vi "TDK工况电流1.vi"() -> ()   [LabVIEW 2020]
uses:
  <vilib>/Utility/file.llb/Read Delimited Spreadsheet (DBL).vi
  <instrlib>/TDK-Lambda G Series/TDK-Lambda G Series.lvlib
panel:
  in  "循环次数":i32
  out "XY Graph":cluster{"Y":dbl[], "Y":dbl[]}[](graph) caption="XY图"
  in  "VISA resource name":refnum<visa-resource-name>
  in  "file path (dialog if empty)":path caption="文件路径 （空时为对话框）"
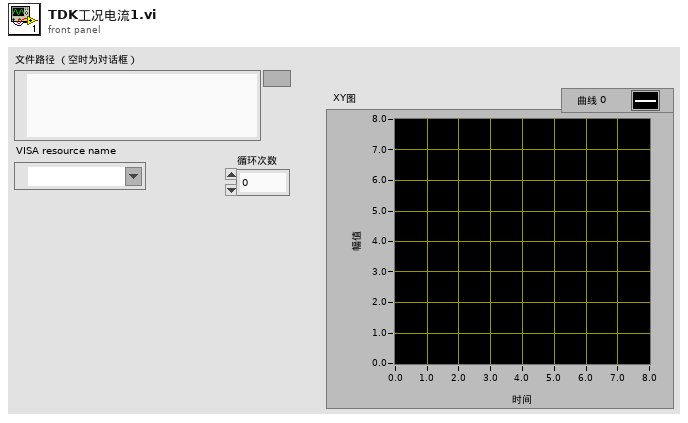
[diagram p1: front panel]
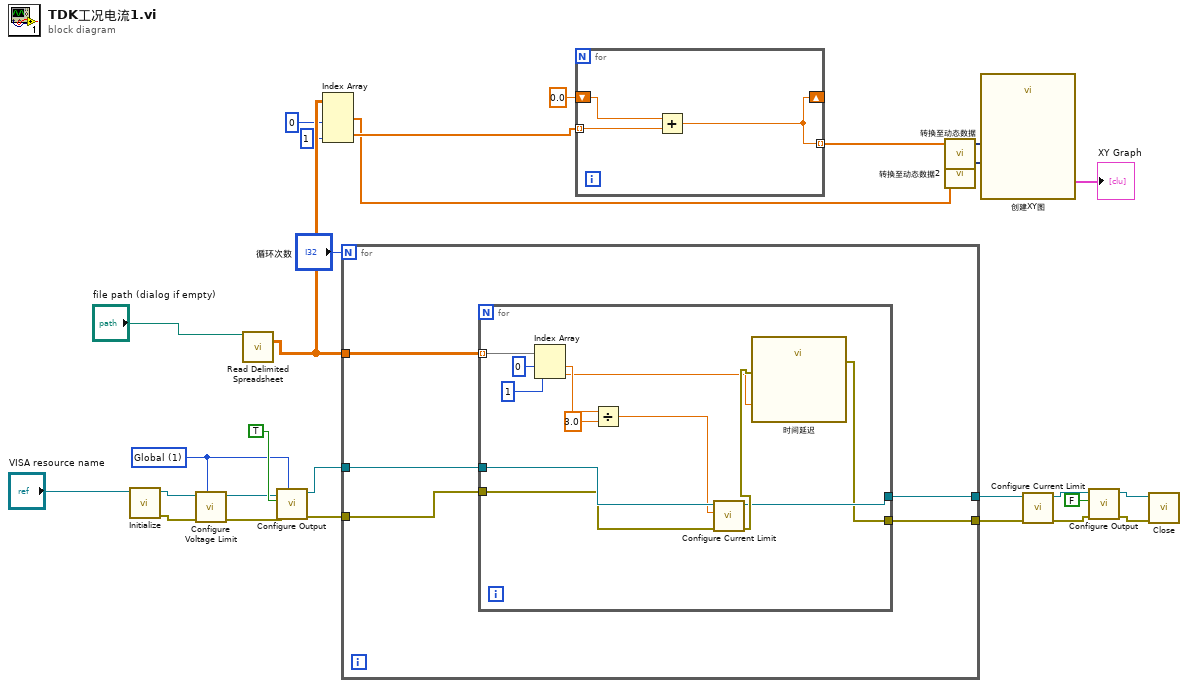
[diagram p0: block diagram]
diagram:
  w23 = u16 1 items=["Single", "Global"] ("Globalize (0: Single)")
  n1 = call <instrlib>:"Initialize.vi"("VISA resource name"="VISA resource name") -> ("error out"=w25:errorcluster, "VISA resource name out"=w22:refnum<visa-resource-name>)  [unwired: 9 in]
  n2 = call <instrlib>:"Configure Voltage Limit.vi"("Globalize (0: Single)"=w23, "error in (no error)"=w25, "VISA resource name"=w22) -> ("error out"=w24:errorcluster, "VISA resource name out"=w21:refnum<visa-resource-name>)  [unwired: 7 in]
  n3 = call-poly <vilib>:"Read Delimited Spreadsheet.vi"("file path (dialog if empty)"="file path (dialog if empty)") -> ("all rows"=w11:dbl[][])  [unwired: 9 in, 5 out]
  n4 = call <instrlib>:"Configure Output.vi"("Globalize (0: Single)"=w23, "error in (no error)"=w24, "Enable Output (False)"=TRUE, "VISA resource name"=w21) -> ("error out"=w19:errorcluster, "VISA resource name out"=w20:refnum<visa-resource-name>)  [unwired: 6 in]
  n5 = Index Array(array=w11, index (col) #1=0 ("禁用的索引 (列)"), index (col) #2=1 ("禁用的索引 (列)")) -> (element #1=w3:dbl[], element #2=w10:dbl[])  [unwired: 2 in]
  n6 = for {
    N: "循环次数" -> [_]
    tunnel: w20 -> [w33]
    tunnel: w19 -> [w32]
    tunnel: w11 -> [w31]
    tunnel: [w30] -> w18
    tunnel: [w29] -> w17
    n7 = for {
      tunnel: w33 -> [w45]
      tunnel: w32 -> [w44]
      tunnel: w31 -> [w43] mode=indexing
      tunnel: [w36] -> w30
      tunnel: [w35] -> w29
      n8 = Index Array(array=w43, index #1=0 ("索引"), index #2=1 ("索引")) -> (element #1=w40:dbl, element #2=w34:dbl)
      n9 = Divide(x=w40, y=3.0) -> (x/y=w38:dbl)
      n10 = call "Configure Current Limit.vi"("error in (no error)"=w44, "Current Limit (0A)"=w38, "VISA resource name"=w45) -> ("error out"=w37:errorcluster, "VISA resource name out"=w36:refnum<visa-resource-name>)  [unwired: 7 in]
      n11 = call "时间延迟"("error in (no error)"=w37, "Delay Time (s)"=w34) -> ("error out"=w35:errorcluster)  [unwired: 9 in]
    }
  }
  n12 = for {
    shift-right: [w46] -> _
    shift-left: 0.0 -> [w48]
    tunnel: w10 -> [w47] mode=indexing
    tunnel: [w46] -> w5 mode=indexing
    n13 = Add(x=w48, y=w47) -> (x+y=w46:dbl)
  }
  n14 = call "转换至动态数据"("Array"=w5) -> ("Dynamic Data Type"=w4:dynamicdata)  [unwired: 3 in]
  n15 = call "转换至动态数据2"("Array"=w3) -> ("Dynamic Data Type"=w2:dynamicdata)  [unwired: 3 in]
  n16 = call "创建XY图"("Y Input"=w2, "X Input"=w4) -> ("XY Graph"=→"XY Graph":cluster{"X":dbl[], "Y":dbl[]}[])  [unwired: 8 in, 1 out]
  n17 = call "Configure Current Limit.vi"("error in (no error)"=w17, "VISA resource name"=w18) -> ("error out"=w14:errorcluster, "VISA resource name out"=w16:refnum<visa-resource-name>)  [unwired: 8 in]
  n18 = call <instrlib>:"Configure Output.vi"("error in (no error)"=w14, "Enable Output (False)"=FALSE, "VISA resource name"=w16) -> ("error out"=w13:errorcluster, "VISA resource name out"=w12:refnum<visa-resource-name>)  [unwired: 7 in]
  n19 = call <instrlib>:"Close.vi"("error in (no error)"=w13, "VISA resource name"=w12) -> ()  [unwired: 9 in, 1 out]
